vi "Frame Get c.vi"(8 "error in (no error)":errorcluster, 11 "IDE simple in":refnum<class "LF2R IDE.lvclass">) -> (0 "error out":errorcluster, 2 "<c> Data":T1, 3 "IDE simple out":refnum<class "LF2R IDE.lvclass">)   [LabVIEW 2018, in "LF2R IDE.lvlib" / "LF2R IDE.lvclass"]
uses:
  LF2R IDE.lvclass
  Frame Analizer/frame c data.ctl
  LF2R IDE.lvclass/LF2R IDE.ctl
  Frame Analizer/Data Parser.lvclass
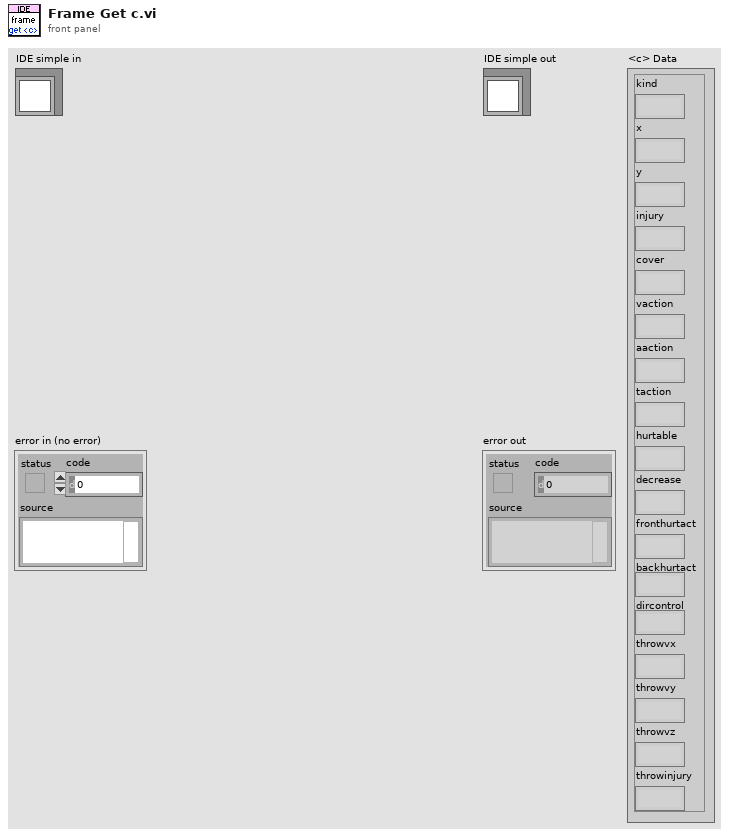
[diagram p1: front panel]
types:
  T1 = typedef "Data Parser.lvclass/frame c data.ctl" = cluster{"kind":string, "x":string, "y":string, "injury":string, "cover":string, "vaction":string, "aaction":string, "taction":string, "hurtable":string, "decrease":string, "fronthurtact":string, "backhurtact":string, "dircontrol":string, "throwvx":string, "throwvy":string, "throwvz":string, "throwinjury":string}
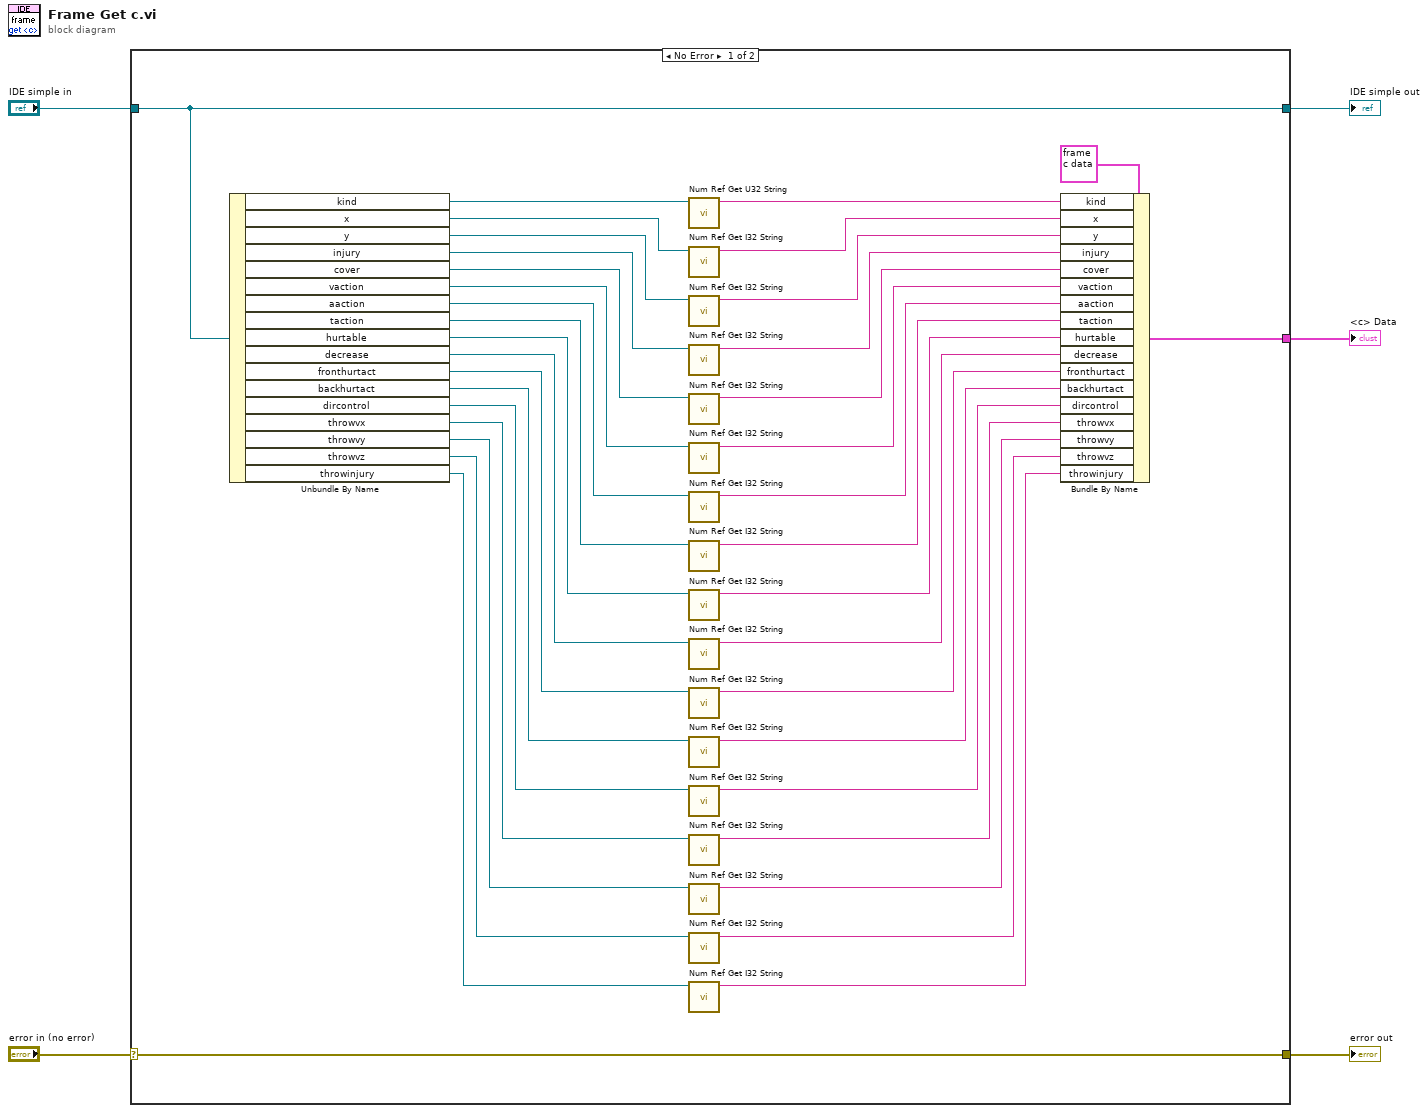
[diagram p0: block diagram]
diagram:
  n1 = case shown="No Error" "error in (no error)" {
    selector: "error in (no error)" -> [w40 w45]
    tunnel: [w40 w45] -> w4
    tunnel: [w43 w44] -> w2
    tunnel: "IDE simple in" -> [w43 w44]
    tunnel: [w42 _] -> w1
    frame No Error {
      n2 = Unbundle By Name(w43) -> ("kind"=w39:refnum<vi>, "x"=w37:refnum<vi>, "y"=w36:refnum<vi>, "injury"=w35:refnum<vi>, "cover"=w34:refnum<vi>, "vaction"=w33:refnum<vi>, "aaction"=w32:refnum<vi>, "taction"=w31:refnum<vi>, "hurtable"=w30:refnum<vi>, "decrease"=w29:refnum<vi>, "fronthurtact"=w28:refnum<vi>, "backhurtact"=w27:refnum<vi>, "dircontrol"=w26:refnum<vi>, "throwvx"=w25:refnum<vi>, "throwvy"=w24:refnum<vi>, "throwvz"=w23:refnum<vi>, "throwinjury"=w22:refnum<vi>)
      n3 = call "Num Ref Get U32 String.vi"("U32 Ref"=w39) -> ("Value string"=w38:string)  [unwired: 9 in, 1 out]
      n4 = call "Num Ref Get I32 String.vi"("I32 Ref"=w37) -> ("Value String"=w21:string)  [unwired: 9 in, 1 out]
      n5 = call "Num Ref Get I32 String.vi"("I32 Ref"=w36) -> ("Value String"=w20:string)  [unwired: 9 in, 1 out]
      n6 = call "Num Ref Get I32 String.vi"("I32 Ref"=w35) -> ("Value String"=w19:string)  [unwired: 9 in, 1 out]
      n7 = call "Num Ref Get I32 String.vi"("I32 Ref"=w34) -> ("Value String"=w18:string)  [unwired: 9 in, 1 out]
      n8 = call "Num Ref Get I32 String.vi"("I32 Ref"=w33) -> ("Value String"=w17:string)  [unwired: 9 in, 1 out]
      n9 = call "Num Ref Get I32 String.vi"("I32 Ref"=w32) -> ("Value String"=w16:string)  [unwired: 9 in, 1 out]
      n10 = call "Num Ref Get I32 String.vi"("I32 Ref"=w31) -> ("Value String"=w15:string)  [unwired: 9 in, 1 out]
      n11 = call "Num Ref Get I32 String.vi"("I32 Ref"=w30) -> ("Value String"=w14:string)  [unwired: 9 in, 1 out]
      n12 = call "Num Ref Get I32 String.vi"("I32 Ref"=w29) -> ("Value String"=w13:string)  [unwired: 9 in, 1 out]
      n13 = call "Num Ref Get I32 String.vi"("I32 Ref"=w28) -> ("Value String"=w12:string)  [unwired: 9 in, 1 out]
      n14 = call "Num Ref Get I32 String.vi"("I32 Ref"=w27) -> ("Value String"=w11:string)  [unwired: 9 in, 1 out]
      n15 = call "Num Ref Get I32 String.vi"("I32 Ref"=w26) -> ("Value String"=w10:string)  [unwired: 9 in, 1 out]
      n16 = call "Num Ref Get I32 String.vi"("I32 Ref"=w25) -> ("Value String"=w9:string)  [unwired: 9 in, 1 out]
      n17 = call "Num Ref Get I32 String.vi"("I32 Ref"=w24) -> ("Value String"=w8:string)  [unwired: 9 in, 1 out]
      n18 = call "Num Ref Get I32 String.vi"("I32 Ref"=w23) -> ("Value String"=w7:string)  [unwired: 9 in, 1 out]
      n19 = call "Num Ref Get I32 String.vi"("I32 Ref"=w22) -> ("Value String"=w6:string)  [unwired: 9 in, 1 out]
      n20 = Bundle By Name(cluster=T1 {"kind"="", "x"="", "y"="", "injury"="", "cover"="", "vaction"="", "aaction"="", "taction"="", "hurtable"="", "decrease"="", "fronthurtact"="", "backhurtact"="", "dircontrol"="", "throwvx"="", "throwvy"="", "throwvz"="", "throwinjury"=""} ("<c> data 2"), "kind"=w38, "x"=w21, "y"=w20, "injury"=w19, "cover"=w18, "vaction"=w17, "aaction"=w16, "taction"=w15, "hurtable"=w14, "decrease"=w13, "fronthurtact"=w12, "backhurtact"=w11, "dircontrol"=w10, "throwvx"=w9, "throwvy"=w8, "throwvz"=w7, "throwinjury"=w6) -> (w42:T1)
    }
    frame Error {
    }
  }
  "error out" <- w4
  "IDE simple out" <- w2
  "<c> Data" <- w1
